vi "Float_to_string.vi"(10 "Array":dbl[](array[numeric]), 11 "Ring":u16(ring) items=["2decimal", "3decimal", "4decimal"]) -> (3 "Array 2":string[](array[string]))   [LabVIEW 2021]
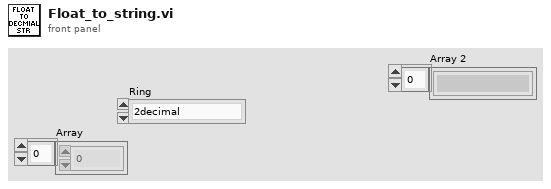
[diagram p1: front panel]
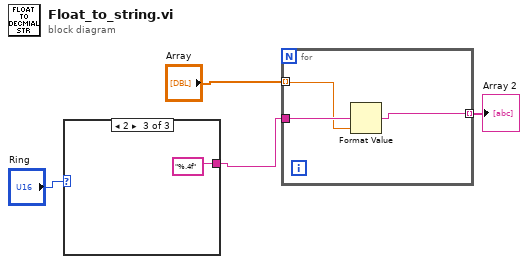
[diagram p0: block diagram]
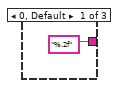
[diagram p2: hidden frame]
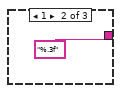
[diagram p3: hidden frame]
diagram:
  n1 = case shown="2" "Ring" {
    tunnel: ["%.2f" "%.3f" "%.4f"] -> w3
    frame 0, Default {
    }
    frame 1 {
    }
    frame 2 {
    }
  }
  n2 = for {
    tunnel: [w10] -> w1 mode=indexing
    tunnel: w3 -> [w9]
    tunnel: "Array" -> [w8] mode=indexing
    n3 = Format Value(format string=w9, value (0)=w8) -> (output string=w10:string)  [unwired: 1 in]
  }
  "Array 2" <- w1
